vi "JKISM+ Duplicate Modules.vi"   [LabVIEW 2014]
uses:
  user.lib/_NEVSTOP/JKI State Machine ++/JKI-State-Machine-Plus.lvlib
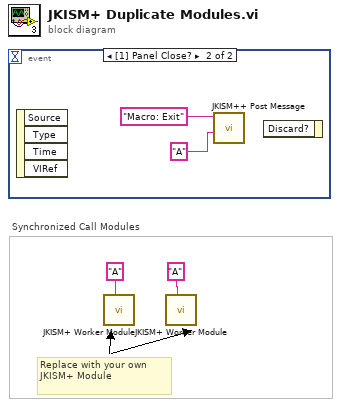
[diagram p0: block diagram]
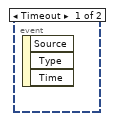
[diagram p2: hidden frame]
diagram:
  # "Synchronized Call Modules"
  # "Replace with your own JKISM+ Module"
  n1 = event shown="[1] Panel Close?" {
    selector: _ -> [_ _]
    dyn-events: _ -> [_ _]
    timeout: _ -> [_ _]
    event Timeout {
      n2 = event-data() -> ()  [unwired: 1 in, 3 out]
    }
    event Panel Close? {
      n3 = event-data() -> ()  [unwired: 1 in, 4 out]
      n4 = call "JKISM++ Post Message.vi"("Dest Module"="A" ("Name"), "States"="Macro: Exit" ("Name")) -> ()  [unwired: 9 in, 1 out]
      n5 = event-data() -> ()  [unwired: 2 in, 1 out]
    }
  }
  n6 = call "JKISM+ Worker Module.vi"("Name(\"\" to use uuid)"="A" ("Name")) -> ()  [unwired: 11 in]
  n7 = call "JKISM+ Worker Module.vi"("Name(\"\" to use uuid)"="A" ("Name")) -> ()  [unwired: 11 in]
